vi "XY Graph Is Grid Hidden.vi"(8 "Error In":errorcluster, 11 "XY Graph Ref":T1) -> (0 "Error Out (dup)":errorcluster, 1 "Hidden Grid(s)":bool, 3 "XY Graph Ref out":T1)   [LabVIEW 2021, in "XY Graph Add-Ons.lvlib"]
uses:
  XY Graph Add-Ons.lvlib
  XY Graph Refnum.ctl
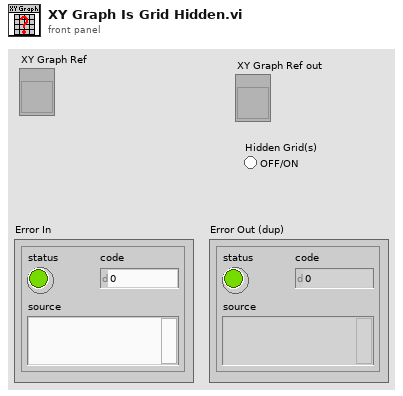
[diagram p1: front panel]
types:
  T1 = typedef "XY Graph Add-Ons.lvlib/XY Graph Refnum.ctl" = refnum<vi>
  T2 = typedef "LVMajorAndMinorColorsTypeDef.ctl" = cluster{"Major Color":u32, "Minor Color":u32}
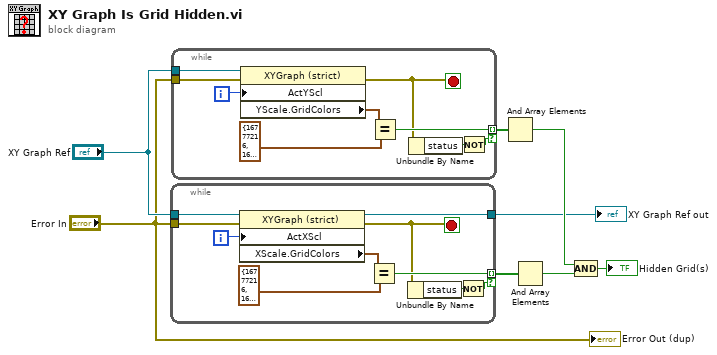
[diagram p0: block diagram]
diagram:
  n1 = while {
    tunnel: "Error In" -> [w17]
    tunnel: [w14] -> w8 mode=indexing if=w10
    tunnel: "XY Graph Ref" -> [w18]
    tunnel: [w9] -> w1
    i -> [w13]
    stop <- w12 stop-if-true
    n2 = property class="XYGraph (strict)"(reference=w18, error in=w17, "ActXScl"=w13) -> (reference out=w9:T1, error out=w12:errorcluster, "XScale.GridColors"=w16:T2)
    n3 = Equal?(x=w16, y=cluster{"Major Color":u32, "Minor Color":u32} {"Major Color"=16777216, "Minor Color"=16777216} ("X Scale.Grid Colors")) -> (x = y?=w14:bool)
    n4 = Unbundle By Name(w12) -> ("status"=w11:bool)
    n5 = Not(x=w11) -> (.not. x?=w10:bool)
  }
  "XY Graph Ref out" <- w1
  n6 = while {
    tunnel: "Error In" -> [w26]
    tunnel: [w23] -> w3 mode=indexing if=w19
    tunnel: "XY Graph Ref" -> [w27]
    i -> [w22]
    stop <- w21 stop-if-true
    n7 = property class="XYGraph (strict)"(reference=w27, error in=w26, "ActYScl"=w22) -> (error out=w21:errorcluster, "YScale.GridColors"=w25:T2)  [unwired: 1 out]
    n8 = Equal?(x=w25, y=cluster{"Major Color":u32, "Minor Color":u32} {"Major Color"=16777216, "Minor Color"=16777216} ("X Scale.Grid Colors")) -> (x = y?=w23:bool)
    n9 = Unbundle By Name(w21) -> ("status"=w20:bool)
    n10 = Not(x=w20) -> (.not. x?=w19:bool)
  }
  n11 = And Array Elements(Boolean array=w3) -> (logical AND=w6:bool)
  n12 = And Array Elements(Boolean array=w8) -> (logical AND=w5:bool)
  n13 = Compound Arithmetic op=AND(w6, w5) -> (→"Hidden Grid(s)":bool)
  "Error Out (dup)" <- "Error In"
